vi "Timeout.vi"(8 "error in":errorcluster, 11 "Loop Data In":T1={"VI Refnum"=refnum, "Timeout"=-1, "Code Data"=[], "Buffer Data"={"Connection ID"=refnum}, "Timer"=4294967295, "Image"=refnum}) -> (0 "error out":errorcluster, 3 "Loop Data Out":T1={"VI Refnum"=refnum, "Timeout"=-1, "Code Data"=[], "Buffer Data"={"Connection ID"=refnum}, "Timer"=4294967295, "Image"=refnum})   [LabVIEW 2016]
uses:
  Data Def/Loop Data.ctl
  Com/Matrix220/Data Def/Com_Matrix220_Buffer Data.ctl
  <vilib>/vision/Image Controls.llb/IMAQ Image.ctl
  <vilib>/picture/picture.llb/imagedata.ctl
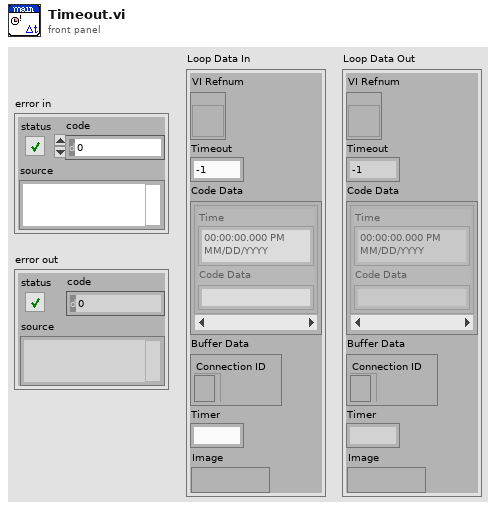
[diagram p1: front panel]
types:
  T1 = typedef "Loop Data.ctl" = cluster{"VI Refnum":refnum<vi>, "Timeout":i32, "Code Data":cluster{"Time":timestamp, "Code Data":string}[], "Buffer Data":T2, "Timer":u32, "Image":T3}
  T2 = typedef "Com_Matrix220_Buffer Data.ctl" = cluster{"Connection ID":refnum<k5>}
  T3 = typedef "IMAQ Image.ctl" = refnum<image>
  T4 = typedef "Com_Matrix220_Message Type.ctl" = enum16{"Unkown", "Ack", "Code", "Image"}
  T5 = typedef "imagedata.ctl" = cluster{"image type":i32, "image depth":i32, "image":u8[], "mask":u8[], "colors":u32[], "Rectangle":cluster{"left":i16, "top":i16, "right":i16, "bottom":i16}}
  T6 = cluster{"seconds since 1Jan1904":timestamp, string}
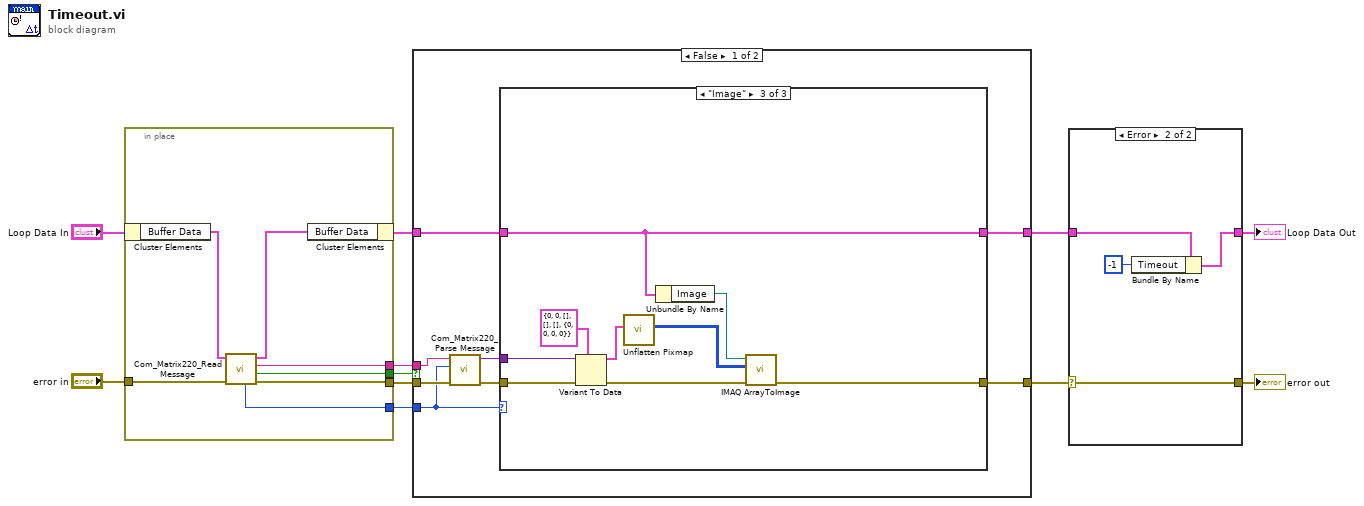
[diagram p0: block diagram]
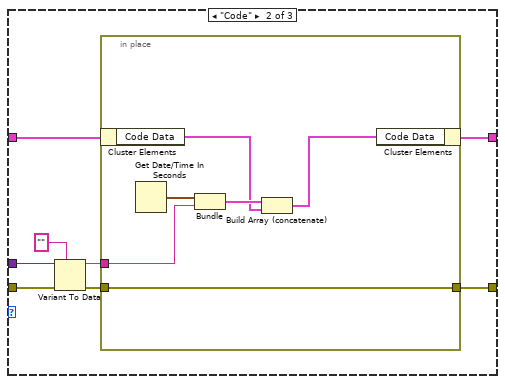
[diagram p3: hidden frame]
diagram:
  n1 = in-place {
    in-place-border: "error in" -> [w16]
    in-place-border: [w15] -> w6
    in-place-border: [w14] -> w7
    in-place-border: [w13] -> w5
    in-place-border: [w12] -> w1
    n2 = in-place-cluster #1("Loop Data In") -> ("Buffer Data"=w18:T2)
    n3 = call "Com_Matrix220_Read Message.vi"("error in"=w16, "Buffer Data In"=w18) -> ("error out"=w15:errorcluster, "Timeout?"=w14:bool, "Message"=w13:string, "Buffer Data Out"=w17:T2, "Message Type"=w12:T4)  [unwired: 5 in]
    n4 = in-place-cluster #1("Buffer Data"=w17) -> (w4:T1)
  }
  n5 = case shown="False" w7 {
    tunnel: w6 -> [w23 w52]
    tunnel: w5 -> [w22 _]
    tunnel: w4 -> [w26 w53]
    tunnel: [w25 w52] -> w3
    tunnel: [w24 w53] -> w2
    tunnel: w1 -> [w21 _]
    frame False {
      n6 = call "Com_Matrix220_Parse Message.vi"("error in"=w23, "Message Type"=w21, "Message"=w22) -> ("error out"=w20:errorcluster, "Variant"=w19:variant)  [unwired: 7 in]
      n7 = case shown="\"Image\"" w21 {
        tunnel: w26 -> [w28 w36 w44]
        tunnel: [w27 w35 w45] -> w25
        tunnel: [w28 w34 w44] -> w24
        tunnel: w20 -> [w27 w33 w51]
        tunnel: w19 -> [_ w32 w50]
        frame "Unkown", Default {
        }
        frame "Code" {
          n8 = Variant To Data(error in=w33, type="", Variant=w32) -> (data=w29:string, error out=w30:errorcluster)
          n9 = in-place {
            in-place-border: w29 -> [w42]
            in-place-border: w30 -> [w37]
            in-place-border: [w37] -> w35
            n10 = in-place-cluster #2(w36) -> ("Code Data"=w39:cluster{"Time":timestamp, "Code Data":string}[])
            n11 = Get Date/Time In Seconds() -> (seconds since 1Jan1904=w41:timestamp)
            n12 = Bundle("seconds since 1Jan1904"=w41, w42) -> (w40:T6)  [unwired: 1 in]
            n13 = Build Array (concatenate)(w40, w39) -> (w38:cluster{"Time":timestamp, "Code Data":string}[])
            n14 = in-place-cluster #2("Code Data"=w38) -> (w34:T1)
          }
        }
        frame "Image" {
          n15 = Variant To Data(error in=w51, type=T5 {"image type"=0, "image depth"=0, "image"=[], "mask"=[], "colors"=[], "Rectangle"={"left"=0, "top"=0, "right"=0, "bottom"=0}} ("Image Data"), Variant=w50) -> (data=w48:T5, error out=w47:errorcluster)
          n16 = call <vilib>:"Unflatten Pixmap.vi"("image data"=w48) -> ("8-bit pixmap"=w43:u8[][])  [unwired: 4 in, 6 out]
          n17 = Unbundle By Name(w44) -> ("Image"=w46:T3)
          n18 = call "IMAQ ArrayToImage"("error in (no error)"=w47, "Image Pixels (U8)"=w43, "Image"=w46) -> ("error out"=w45:errorcluster)  [unwired: 7 in, 1 out]
        }
      }
    }
    frame True {
    }
  }
  n19 = case shown="Error" w3 {
    selector: w3 -> [w54 w56]
    tunnel: w2 -> [w55 w59]
    tunnel: [w55 w57] -> w9
    tunnel: [w54 w56] -> w8
    frame No Error {
    }
    frame Error {
      n20 = Bundle By Name(cluster=w59, "Timeout"=-1) -> (w57:T1)
    }
  }
  "error out" <- w8
  "Loop Data Out" <- w9
